vi "_ManagerOpen.vi"(8 "error in":errorcluster, 11 "Device In":u64) -> (0 "error out":errorcluster, 3 "Device Out":u64)   [LabVIEW 2012, in "Phidget Manager.lvlib"]
doc: "Opens a Public"
uses:
  <instrlib>/Phidgets/Phidget Manager/Phidget Manager.lvlib
  <instrlib>/Phidgets/Phidget Common/Phidget Common.lvlib
  phidget22.dll
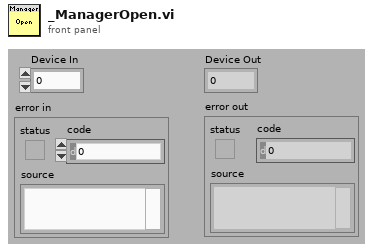
[diagram p1: front panel]
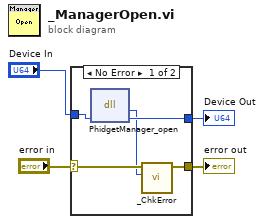
[diagram p0: block diagram]
diagram:
  n1 = case shown="No Error" "error in" {
    selector: "error in" -> [w7 w11]
    tunnel: [w5 w11] -> w3
    tunnel: [w9 w10] -> w2
    tunnel: "Device In" -> [w8 w10]
    frame No Error {
      n2 = dll-call lib="phidget22.dll" fn="PhidgetManager_open"("phid"=w8) -> ("return type"=w6:i32, "phid"=w9:u64)  [unwired: 3 in, 2 out]
      n3 = call <instrlib>:"_ChkError.vi"("Return Code"=w6, "error in (no error)"=w7) -> ("error out"=w5:errorcluster)  [unwired: 9 in]
    }
    frame Error {
    }
  }
  "error out" <- w3
  "Device Out" <- w2
